vi "LaunchUserSystem.vi"   [LabVIEW 2015]
uses:
  Member_Actor/Member_Actor/Member_Actor.lvclass
  <vilib>/ActorFramework/Actor/Actor.lvclass
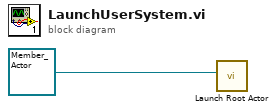
[diagram p0: block diagram]
diagram:
  n1 = call <vilib>:"Launch Root Actor.vi"("Actor"=refnum<class "Member_Actor.lvclass"> refnum ("Member_Actor.lvlib:Member_Actor.lvclass")) -> ()  [unwired: 9 in, 2 out]
